vi "Alex_write_command_and_read.vi"(0 "VISA resource name":refnum<visa-resource-name>, 1 "Wait before read (0ms)":u32, 2 "Command":string, 3 "Bytes to read (100)":u32=100, 5 "error in (no error)":errorcluster) -> (7 "Returned string":string)   [LabVIEW 2017]
uses:
  Newport ESP301/Newport ESP301.lvlib
panel:
  in  "ID Query (True)":bool=TRUE
  in  "Reset (False)":bool
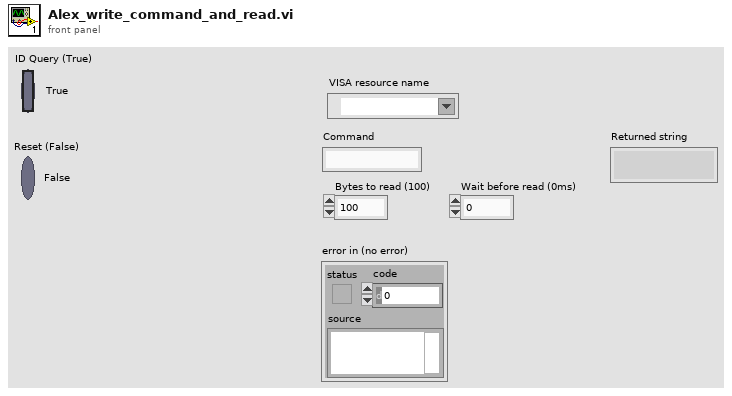
[diagram p1: front panel]
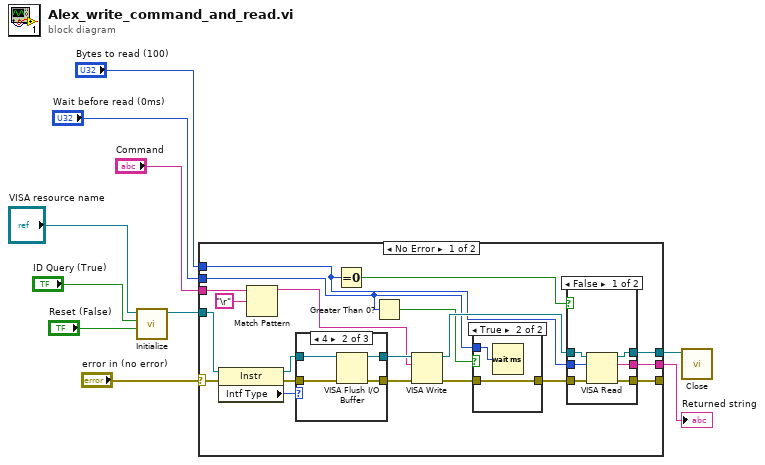
[diagram p0: block diagram]
diagram:
  n1 = call "Initialize.vi"("VISA resource name"="VISA resource name", "ID Query (True)"="ID Query (True)", "Reset (False)"="Reset (False)") -> ("VISA resource name out"=w4:refnum<visa-resource-name>)  [unwired: 6 in, 1 out]
  n2 = case shown="No Error" "error in (no error)" {
    selector: "error in (no error)" -> [w15 w51]
    tunnel: [w30 w51] -> _
    tunnel: w4 -> [w17 w50]
    tunnel: [w28 w50] -> w1
    tunnel: "Command" -> [w13 _]
    tunnel: "Bytes to read (100)" -> [w20 _]
    tunnel: [w27 _] -> w7
    tunnel: "Wait before read (0ms)" -> [w22 _]
    frame No Error {
      n3 = property class="Instr"(reference=w17, error in=w15) -> (reference out=w16:refnum<visa-resource-name>, error out=w14:errorcluster, "Intf Type"=w18:u16)
      n4 = Match Pattern(string=w13, regular expression="\r") -> (before substring=w11:string)  [unwired: 4 out]
      n5 = case shown="4" w18 {
        tunnel: w16 -> [w32 w34 w38]
        tunnel: [w32 w33 w38] -> w26
        tunnel: w14 -> [w31 w36 w37]
        tunnel: [w31 w35 w37] -> w25
        frame 1 {
        }
        frame 4 {
          n6 = VISA Flush I/O Buffer(VISA resource name=w34, error in (no error)=w36) -> (VISA resource name out=w33:refnum<visa-resource-name>, error out=w35:errorcluster)  [unwired: 1 out]
        }
        frame Default {
        }
      }
      n7 = Equal To 0?(x=w20) -> (x = 0?=w19:bool)
      n8 = Greater Than 0?(x=w22) -> (x > 0?=w21:bool)
      n9 = VISA Write(VISA resource name=w26, write buffer=w11, error in (no error)=w25) -> (VISA resource name out=w29:refnum<visa-resource-name>, error out=w24:errorcluster)  [unwired: 1 out]
      n10 = case shown="True" w21 {
        tunnel: w24 -> [w47 w49]
        tunnel: [w47 w49] -> w23
        tunnel: w22 -> [_ w48]
        frame False {
        }
        frame True {
          n11 = Wait (ms)(milliseconds to wait=w48) -> ()  [unwired: 1 out]
        }
      }
      n12 = case shown="False" w19 {
        tunnel: [w44 w46] -> w30
        tunnel: w29 -> [w43 w45]
        tunnel: [w42 w45] -> w28
        tunnel: w20 -> [w41 _]
        tunnel: [w40 _] -> w27
        tunnel: w23 -> [w39 w46]
        frame False {
          n13 = VISA Read(VISA resource name=w43, byte count=w41, error in (no error)=w39) -> (VISA resource name out=w42:refnum<visa-resource-name>, read buffer=w40:string, error out=w44:errorcluster)  [unwired: 1 out]
        }
        frame True {
        }
      }
    }
    frame Error {
    }
  }
  "Returned string" <- w7
  n14 = call "Close.vi"("VISA resource name"=w1) -> ()  [unwired: 10 in, 1 out]
